vi "SwerveJoystickRotationScaling.vi"(3 "Raw Rotation Joystick":dbl, 5 "Rotation Scaling":dbl(slide)=2.0 min=1.0 max=4.0 scale=1.0..4.0, 6 "Rotation Deadband":dbl(slide)=0.05 min=0.0 max=0.4 scale=0.0..0.4) -> (0 "Scaled Rotation Joystick":dbl, 2 "Out of Deadband":bool)   [LabVIEW 2019]
doc: "Applies a deadband and nonlinear scaling to the rotation axis of a swerve drive."
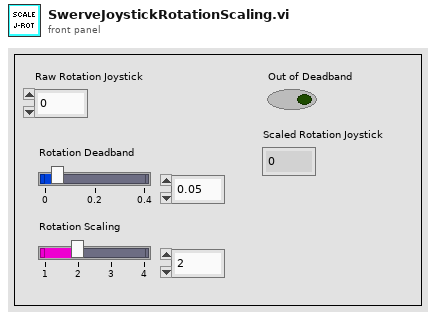
[diagram p1: front panel]
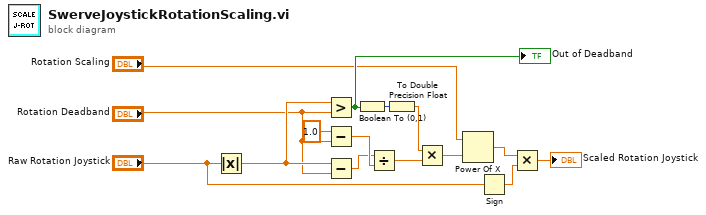
[diagram p0: block diagram]
diagram:
  n1 = Absolute Value(x="Raw Rotation Joystick") -> (abs(x)=w11:dbl)
  n2 = Greater?(x=w11, y="Rotation Deadband") -> (0:w12:bool)
  "Out of Deadband" <- w12
  n3 = Subtract(x=1.0, y="Rotation Deadband") -> (x-y=w7:dbl)
  n4 = Subtract(x=w11, y="Rotation Deadband") -> (x-y=w5:dbl)
  n5 = Boolean To (0,1)(Boolean=w12) -> (0, 1=w3:i16)
  n6 = Divide(x=w5, y=w7) -> (x/y=w8:dbl)
  n7 = To Double Precision Float(number=w3) -> (double precision float=w4:dbl)
  n8 = Multiply(x=w4, y=w8) -> (x*y=w14:dbl)
  n9 = Power Of X(1:w14, 2:"Rotation Scaling") -> (0:w15:dbl)
  n10 = Sign(1:"Raw Rotation Joystick") -> (0:w10:dbl)
  n11 = Multiply(x=w15, y=w10) -> (x*y=→"Scaled Rotation Joystick":dbl)
